vi "asset.links.to_json.vi"(8 "error in":errorcluster, 10 "Links":T1) -> (0 "error out":errorcluster, 2 "json":string)   [LabVIEW 2020, in "Nominal Client.lvclass"]
uses:
  Nominal Client.lvclass
  links.ctl
  01dcef65-c848-435e-b82c-8c09c626b1d5.vi
  5aca689d-ef0c-4f78-ba98-68a9845d9c34.vi
  <vilib>/JDP Science/JSONtext/Variant to JSON Text.vi
  <vilib>/JDP Science/JSONtext/support/Format JSON Object.vi
  <vilib>/JDP Science/JSONtext/support/Format JSON Array Text.vi
  <vilib>/JDP Science/JSONtext/LVClass Serializer/JSONtext LVClass Serializer.lvclass
  <vilib>/JDP Science/JSONtext/JSONtext.lvlib
  nominal types/dataScope/dataScopes.lvlib
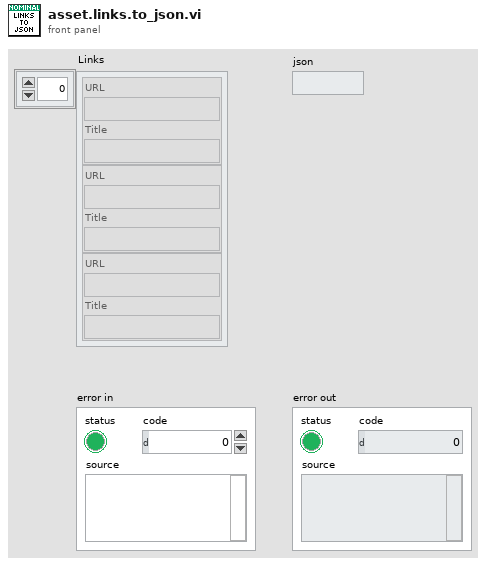
[diagram p1: front panel]
types:
  T1 = typedef "dataScopes.lvlib/links.ctl" = cluster{"URL":string, "Title":string}[]
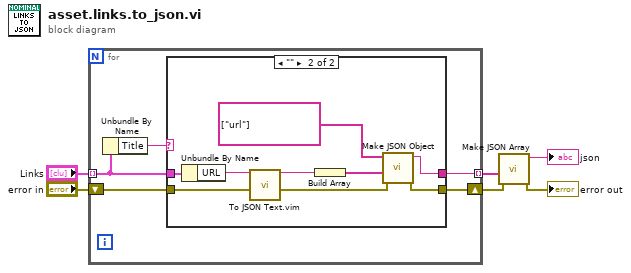
[diagram p0: block diagram]
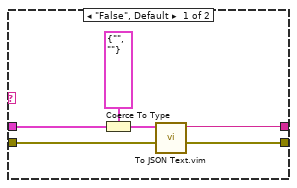
[diagram p2: hidden frame]
diagram:
  n1 = for {
    tunnel: "Links" -> [w11] mode=indexing
    tunnel: [w9] -> w5 mode=indexing
    shift-right: [w8] -> w2
    shift-left: "error in" -> [w7]
    n2 = Unbundle By Name(w11) -> ("Title"=w10:string)
    n3 = case shown="\"\"" w10 {
      tunnel: w11 -> [w15 w22]
      tunnel: [w14 w23] -> w9
      tunnel: [w13 w18] -> w8
      tunnel: w7 -> [w12 w20]
      frame "False", Default {
        n4 = Coerce To Type(0:w15, 1:cluster{"url":string, "title":string} {"url"="", "title"=""} ("type")) -> (2:w17:cluster{"url":string, "title":string})
        n5 = call "To JSON Text.vim"("error in (no error)"=w12, "Anything"=w17) -> ("error out"=w13:errorcluster, "<JSON>"=w14:string)  [unwired: 8 in]
      }
      frame "" {
        n6 = Unbundle By Name(w22) -> ("URL"=w21:string)
        n7 = call "To JSON Text.vim"("error in (no error)"=w20, "Anything"=w21) -> ("error out"=w19:errorcluster, "<JSON>"=w26:string)  [unwired: 8 in]
        n8 = Build Array(w26) -> (w25:string[])
        n9 = call <vilib>:"Make JSON Object.vi"("error in (no error)"=w19, "JSON Items"=w25, "Item Names"=string[] ["url"]) -> ("error out"=w18:errorcluster, "<JSON>"=w23:string)  [unwired: 7 in]
      }
    }
  }
  n10 = call <vilib>:"Make JSON Array.vi"("error in (no error)"=w2, "JSON Elements"=w5) -> ("error out"=→"error out":errorcluster, "<JSON>"=→"json":string)  [unwired: 8 in]
